vi "Thermistor Read.vi"(8 "Error In":errorcluster, 9 "Units (C)":T2, 10 "Thermistor Configuration":T1={"Thermistor AI Pin (0)"=0, "Paired Resistance (10K Ohms)"=10000.0, "Vcc (5 v)"=5.0}, 11 "ChipKit Resource":T3={"COM Port"="COM11", "Board Type"=enum."ChipKit uC32", "Connection Type"=enum."USB / Serial", "Baud Rate (115200)"=15, "Bytes Per Packet (15)"=15}) -> (0 "Error Out":errorcluster, 2 "Temperature":dbl, 3 "ChipKit Resource":T3={"COM Port"="COM11", "Board Type"=enum."ChipKit uC32", "Connection Type"=enum."USB / Serial", "Baud Rate (115200)"=15, "Bytes Per Packet (15)"=15})   [LabVIEW 2011, in "LabVIEW Interface for ChipKit.lvlib"]
doc: "Read the temperature from a thermistor. Thermistor must be used in a voltage divider with a paired resistance. The paired resistance is user selectable however a value of 10K Ohms is recommended."
uses:
  LabVIEW Interface for ChipKit.lvlib
  Private/Type Defs/Chipkit Resource.ctl
  Private/Type Defs/Board Type.ctl
  Private/Type Defs/Connection Type.ctl
  Private/Type Defs/Temperature Units.ctl
  Private/Type Defs/Thermistor Configuration.ctl
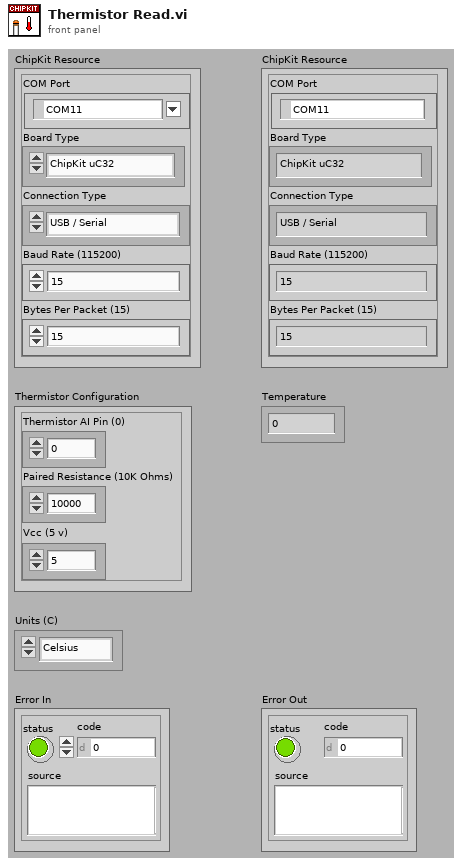
[diagram p1: front panel]
types:
  T1 = typedef "LabVIEW Interface for ChipKit.lvlib/Thermistor Configuration.ctl" = cluster{"Thermistor AI Pin (0)":u8, "Paired Resistance (10K Ohms)":dbl, "Vcc (5 v)":dbl}
  T2 = typedef "LabVIEW Interface for ChipKit.lvlib/Temperature Units.ctl" = enum16{"Celsius", "Fahrenheit", "Kelvin", "Rankine"}
  T3 = typedef "LabVIEW Interface for ChipKit.lvlib/Chipkit Resource.ctl" = cluster{"COM Port":refnum<visa-resource-name>, "Board Type":T4, "Connection Type":T5, "Baud Rate (115200)":u32, "Bytes Per Packet (15)":u32}
  T4 = typedef "LabVIEW Interface for ChipKit.lvlib/Board Type.ctl" = enum16{"ChipKit uC32", "ChipKit Uno32", "ChipKit Max32"}
  T5 = typedef "LabVIEW Interface for ChipKit.lvlib/Connection Type.ctl" = enum8{"USB / Serial", "XBEE", "BlueSmirf (Bluetooth)"}
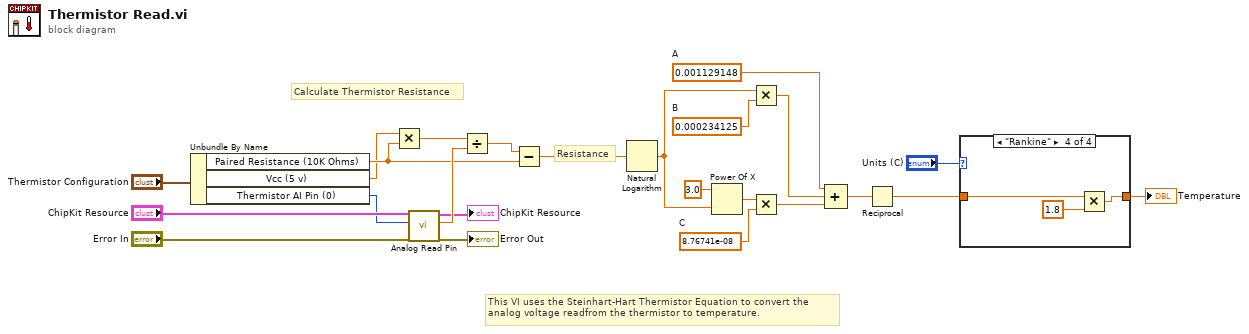
[diagram p0: block diagram]
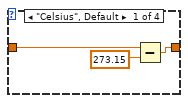
[diagram p2: hidden frame]
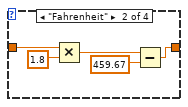
[diagram p3: hidden frame]
diagram:
  w18 = 8.76741e-08  # C
  w15 = 0.001129148  # A
  w20 = 0.000234125  # B
  # "Resistance"
  # "This VI uses the Steinhart-Hart Thermistor Equation to convert the \nanalog voltage readfrom the thermistor to temperature."
  # "Calculate Thermistor Resistance"
  n1 = Unbundle By Name("Thermistor Configuration") -> ("Paired Resistance (10K Ohms)"=w2:dbl, "Vcc (5 v)"=w1:dbl, "Thermistor AI Pin (0)"=w3:u8)
  n2 = Multiply(x=w1, y=w2) -> (x*y=w24:dbl)
  n3 = call "Analog Read Pin.vi"("Error In"="Error In", "Analog Pin"=w3, "ChipKit Resource"="ChipKit Resource") -> ("Error Out"=→"Error Out":errorcluster, "Voltage"=w23:dbl, "ChipKit Resource"=→"ChipKit Resource":T3)  [unwired: 6 in]
  n4 = Divide(x=w24, y=w23) -> (x/y=w22:dbl)
  n5 = Subtract(x=w22, y=w2) -> (x-y=w21:dbl)
  n6 = Natural Logarithm(1:w21) -> (0:w8:dbl)
  n7 = Power Of X(1:w8, 2:3.0 ("x")) -> (0:w19:dbl)
  n8 = Multiply(x=w8, y=w20) -> (x*y=w16:dbl)
  n9 = Multiply(x=w19, y=w18) -> (x*y=w17:dbl)
  n10 = Compound Arithmetic op=ADD(w15, w16, w17) -> (w14:dbl)
  n11 = Reciprocal(x=w14) -> (1/x=w13:dbl)
  n12 = case shown="\"Rankine\"" "Units (C)" {
    tunnel: w13 -> [w27 w32 w33 w34]
    tunnel: [w25 w28 w33 w36] -> w7
    frame "Celsius", Default {
      n13 = Subtract(x=w27, y=273.15) -> (x-y=w25:dbl)
    }
    frame "Fahrenheit" {
      n14 = Multiply(x=w32, y=1.8) -> (x*y=w30:dbl)
      n15 = Subtract(x=w30, y=459.67) -> (x-y=w28:dbl)
    }
    frame "Kelvin" {
    }
    frame "Rankine" {
      n16 = Multiply(x=w34, y=1.8 ("x")) -> (x*y=w36:dbl)
    }
  }
  "Temperature" <- w7
